vi "Get Configuration.vi"(8 "error in":errorcluster, 11 "Configuration in":refnum<class "Configuration.lvclass">) -> (0 "error out":errorcluster, 2 "Configuration":T1, 3 "Configuration out":refnum<class "Configuration.lvclass">)   [LabVIEW 2020, in "Performance Monitor UI.lvlib" / "Configuration.lvclass"]
doc: "____\nPeloton Config 2.0.0.6\nCopyright (c) 2024, Peloton"
uses:
  Configuration.lvclass
  Configuration--cluster.ctl
  Configuration.lvclass/Configuration.ctl
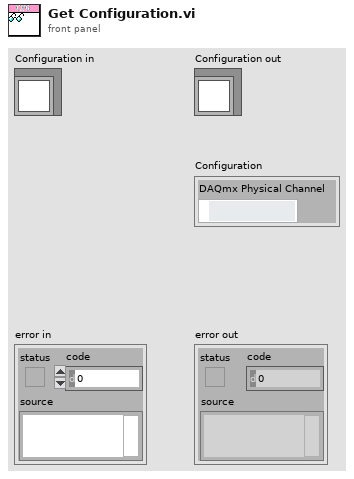
[diagram p1: front panel]
types:
  T1 = typedef "Performance Monitor UI.lvlib/Configuration.lvclass/Configuration--cluster.ctl" = cluster{"DAQmx Physical Channel":tag}
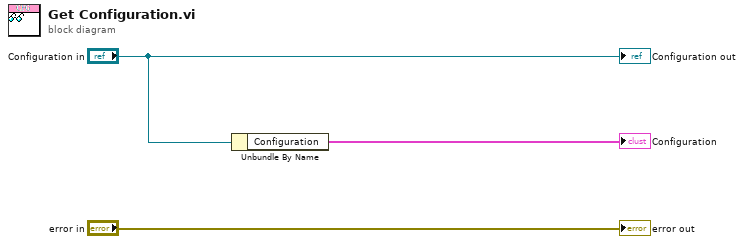
[diagram p0: block diagram]
diagram:
  n1 = Unbundle By Name("Configuration in") -> ("Configuration"=→"Configuration":T1)
  "error out" <- "error in"
  "Configuration out" <- "Configuration in"
